vi "FFT.vi"() -> ()   [LabVIEW 2020]
uses:
  <vilib>/rvi/Analysis/measure/FFT/simModelSupport/niFPGA FFT Outside SCTL Sim Properties.ctl
  <vilib>/rvi/Analysis/measure/FFT/simModelSupport/niFPGA FFT Sim Types.ctl
  <vilib>/rvi/Analysis/measure/FFT/simModelSupport/niFpgaFFTSimArithmeticProperties.ctl
  <vilib>/rvi/Analysis/measure/FFT/simModelSupport/niFpgaFFTSimDfxp.ctl
  <vilib>/fxp/LVFixedPointQuantizationPolicyTypeDef.ctl
  <vilib>/rvi/FXPMathLib/FxpSinAndCos/subVIs/nifxpmath_SinAndCos_SimConfig.ctl
  <vilib>/rvi/DataTransferAndStorage/Container/Common/niFpgaContainerGetUniqueNameForEmu.vi
  <vilib>/rvi/DataTransferAndStorage/Container/Common/niFpgaContainerSetEmuInfo.vi
  <vilib>/rvi/eio/common/nirviEmuReportErrorAndStop.vi
  <vilib>/rvi/interface/RandomDataEmulation/niFpgaRandomDataHandleErrors.vi
  <vilib>/rvi/DataTransferAndStorage/Container/Common/niFpgaContainerExecOnDevCompGetState.vi
  <vilib>/rvi/Emulation/niFpgaEmulationIsFPGAContextNoSignature.vi
  <vilib>/rvi/Emulation/niFpgaSctlEmulationGetInTimedLoop.vi
  <vilib>/rvi/errors/niFpgaSetErrorForExecOnDevCompSimple.vi
  <vilib>/rvi/FIFO/Fifo_Resource/nirvififoEmulationSetSize.vi
  <vilib>/rvi/FIFO/Fifo_Resource/nirviFifoEmulationQueueMgr.vi
  <instcachedir>/0/nirviFifoEmulationQueueMgr_E5CAEC123FF24DC58D834DCA3CDAA9B5.lvgen/nirviFifoEmulationQueueMgr_E5CAEC123FF24DC58D834DCA3CDAA9B5_008.vi
  <vilib>/rvi/FIFO/Fifo_Resource/nirvififoEmulationDetermineInputValidOut.vi
  <vilib>/rvi/FIFO/Fifo_Resource/nirvififoEmulationCreateLock.vi
  <vilib>/rvi/Emulation/niFpgaProcessEmulError.vi
  <vilib>/rvi/FIFO/Fifo_Resource/nirvififoEmulationObtainLock.vi
  <vilib>/rvi/FIFO/Fifo_Resource/nirvififoEmulationReleaseLock.vi
  <vilib>/rvi/occurrence/nirviWaitOnOccurrenceBase.vi
  <vilib>/rvi/errors/nirviReportUnexpectedCaseInternalError.vi
  <vilib>/rvi/errors/nirviReportUnexpectedCaseInternalError (U32).vi
  <vilib>/Utility/error.llb/Clear Errors.vi
  <vilib>/rvi/Emulation/niFpgaGetClockAttributes.vi
  <vilib>/rvi/Emulation/niFpgaEmulationReportErrorSimple.vi
  <vilib>/rvi/Analysis/measure/FFT/simModelSupport/niFpgaFFTSimModelOutsideSCTLCore.vi
  <instcachedir>/0/nirviFifoEmulationQueueMgr_E5CAEC123FF24DC58D834DCA3CDAA9B5.lvgen/nirviFifoEmulationQueueMgr_E5CAEC123FF24DC58D834DCA3CDAA9B5_004.vi
  <vilib>/rvi/FXPMathLib/FxpSinAndCos/simVIs/DllFxpSinAndCosTemp_sub.vi
  <vilib>/rvi/Emulation/niFpgaCriticalErrorInLSC.vi
  <vilib>/rvi/LocalResourceManager/LocalResourceManager.xnode
  <vilib>/rvi/DataTransferAndStorage/Container/XNode/niFpgaContainer.xnode
  <vilib>/rvi/interface/RandomDataEmulation/nirviRandomDataFpgaReadWriteTemplate.vi
  <vilib>/rvi/FIFO/Fifo_Resource/niFpgaFifoEmulationRefIn.vi
  <vilib>/rvi/Analysis/measure/FFT/XNode/niFpgaFFT.xnode
  <vilib>/rvi/FXPMathLib/FxpSinAndCos/XNode/nifxpmath_SinAndCos.xnode
panel:
  out "Numeric 3":i32
  out "Numeric":i32
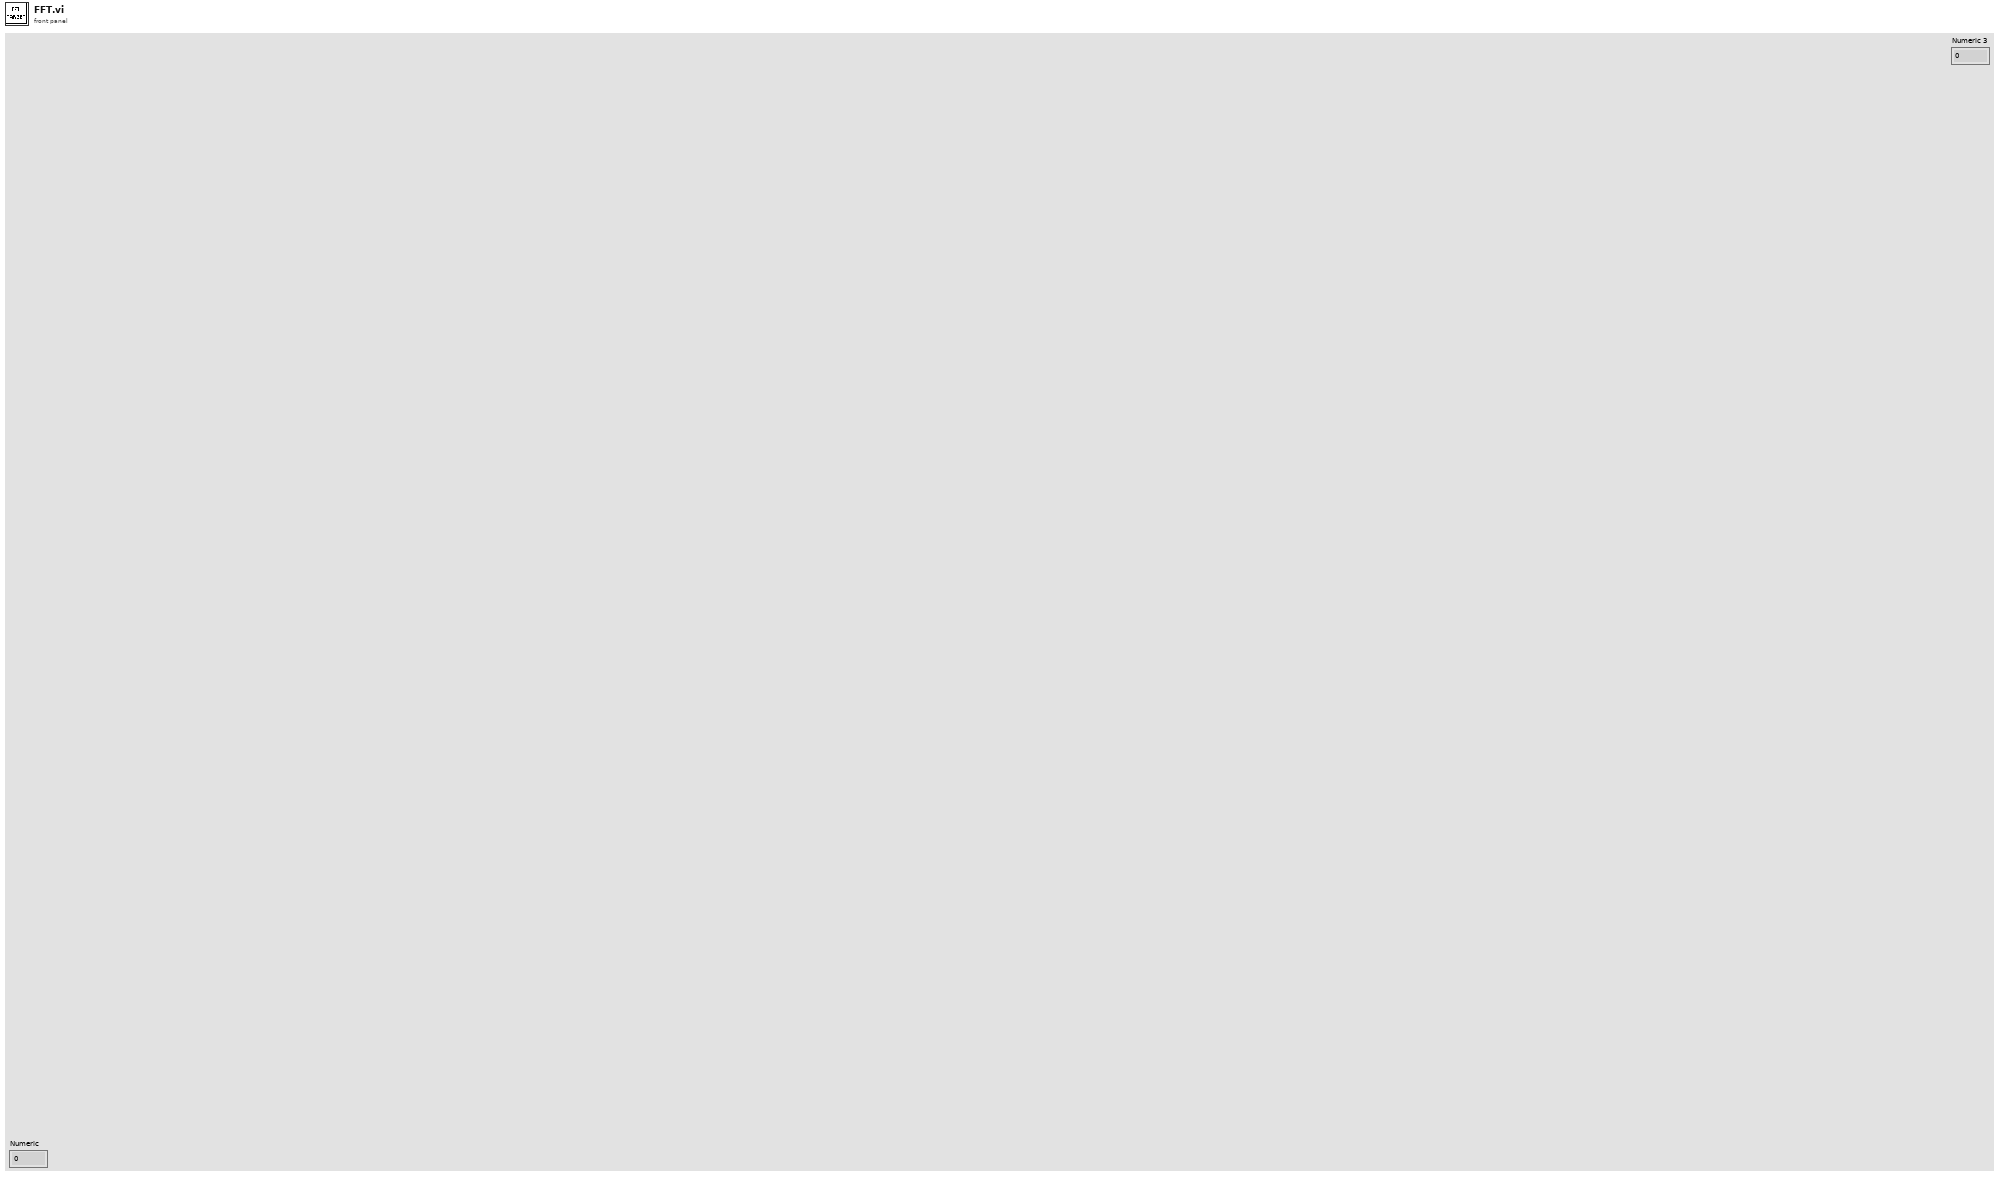
[diagram p1: front panel]
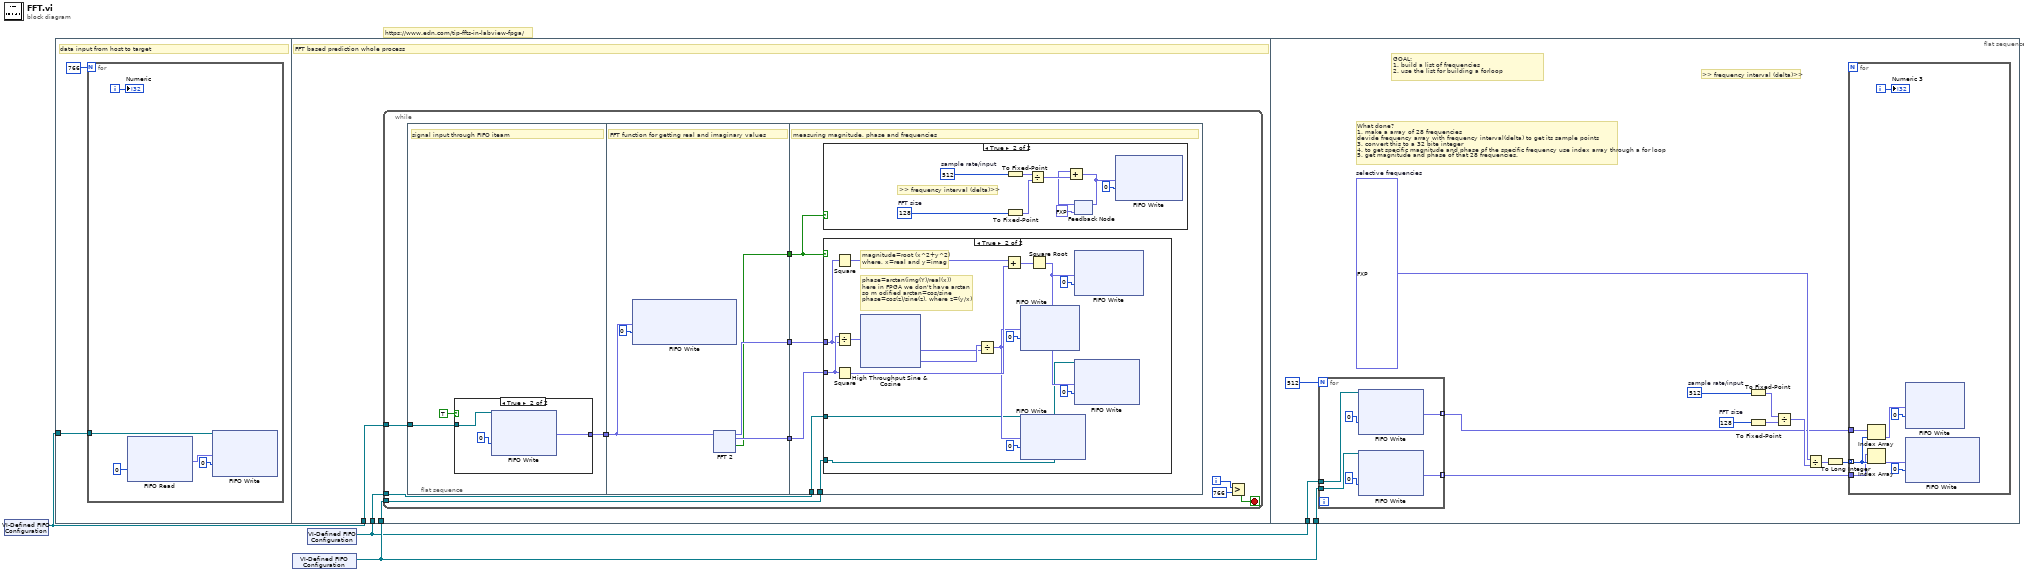
[diagram p0: block diagram]
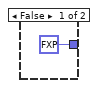
[diagram p2: hidden frame]
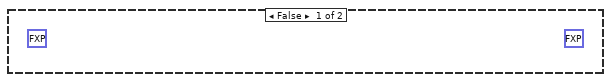
[diagram p4: hidden frame]
diagram:
  # "https://www.edn.com/tip-ffts-in-labview-fpga/"
  n1 = xnode "VI-Defined FIFO Configuration"() -> ("FIFO Out"=w3:refnum<k21>)
  n2 = flat-sequence {
    tunnel: w3 -> [w5]
    tunnel: w3 -> [w13]
    tunnel: w2 -> [w12]
    tunnel: w1 -> [w11]
    tunnel: w2 -> [w117]
    tunnel: w1 -> [w116]
    frame #0 {
      # "data input from host to target"
      n3 = for {
        N: 766 -> [_]
        tunnel: w5 -> [w9]
        i -> [w6]
        n4 = xnode ("FIFO Read")("Timeout"=0) -> ("Element"=w7:fxp<+/-,24,7>)  [unwired: 1 in, 2 out]
        n5 = xnode ("FIFO Write")("Element"=w7, "Timeout"=0, "FIFO In"=w9) -> ()  [unwired: 2 out]
        "Numeric" <- w6
      }
    }
    frame #1 {
      # "FFT based prediction whole process"
      n6 = while {
        tunnel: w13 -> [w22]
        tunnel: w12 -> [w15]
        tunnel: w11 -> [w14]
        i -> [w21]
        stop <- w16 stop-if-true
        n7 = flat-sequence {
          tunnel: w22 -> [w26]
          tunnel: [w24] -> w20
          tunnel: w20 -> [w35]
          tunnel: [w34] -> w19
          tunnel: [w33] -> w18
          tunnel: [w32] -> w17
          tunnel: w19 -> [w59]
          tunnel: w18 -> [w58]
          tunnel: w17 -> [w60]
          tunnel: w15 -> [w57]
          tunnel: w14 -> [w56]
          frame #0 {
            # "signal input through FIFO iteam"
            n8 = case shown="True" TRUE {
              tunnel: w26 -> [_ w30]
              tunnel: [fxp<+/-,24,7> 0.0 ("Element") w28] -> w24
              frame False {
              }
              frame True {
                n9 = xnode ("FIFO Write")("Timeout"=0, "FIFO In"=w30) -> ("Element"=w28:fxp<+/-,24,7>)  [unwired: 2 out]
              }
            }
          }
          frame #1 {
            # "FFT function for getting real and imaginary values"
            n10 = xnode ("FIFO Write")("Element"=w35, "Timeout"=0) -> ()  [unwired: 1 in, 2 out]
            n11 = xnode ("FFT 2")("real data in"=w35) -> ("real data out"=w34:fxp<+/-,32,15>, "imaginary data out"=w33:fxp<+/-,32,15>, "output valid"=w32:bool)  [unwired: 2 in, 1 out]
          }
          frame #2 {
            # "measuring magnitude, phase and frequencies"
            n12 = case shown="True" w60 {
              frame False {
              }
              frame True {
                w61 = 512  # sample rate/input
                w62 = 128  # FFT size
                # ">> frequency interval (delta)>>"
                n13 = To Fixed-Point(number=w61) -> (fixed-point=w64:fxp<+/-,32,32>)  [unwired: 1 in]
                n14 = To Fixed-Point(number=w62) -> (fixed-point=w63:fxp<+/-,32,32>)  [unwired: 1 in]
                n15 = Divide(x=w64, y=w63) -> (x/y=w68:fxp<+/-,32,16>)
                n16 = feedback #1(fxp<+/-,32,16> 0.0) -> (w66:fxp<+/-,32,16>)
                n17 = Add(x=w66, y=w68) -> (x+y=w67:fxp<+/-,32,16>)
                n18 = feedback-in #1(w67) -> ()
                n19 = xnode ("FIFO Write")("Element"=w67, "Timeout"=0) -> ()  [unwired: 1 in, 2 out]
              }
            }
            n20 = case shown="True" w60 {
              tunnel: w58 -> [_ w85]
              tunnel: w59 -> [_ w84]
              tunnel: w57 -> [_ w74]
              tunnel: w56 -> [_ w70]
              frame False {
                (unwired) fxp<+/-,32,16> 0.0
                (unwired) fxp<+/-,32,16> 0.0
              }
              frame True {
                # "magnitude=root (x^2+y^2)\nwhere, x=real and y=imag"
                # "phase=arctan(img(Y)/real(x))\nhere in FPGA we don't have arctan\nso m odified arctan=cos/sine\nphase=cos(z)/sine(z), where z=(y/x)"
                n21 = Square(x=w84) -> (x^2=w79:fxp<+,63,29>)
                n22 = Divide(x=w85, y=w84) -> (x/y=w77:fxp<+/-,32,16>)
                n23 = Square(x=w85) -> (x^2=w73:fxp<+,63,29>)
                n24 = xnode "High Throughput Sine & Cosine"("x (pi)"=w77) -> ("sin(x)"=w80:fxp<+/-,32,2>, "cos(x)"=w81:fxp<+/-,32,2>)
                n25 = Divide(x=w81, y=w80) -> (x/y=w72:fxp<+/-,32,16>)
                n26 = Add(x=w79, y=w73) -> (x+y=w78:fxp<+,64,30>)
                n27 = xnode ("FIFO Write")("Element"=w72, "Timeout"=0) -> ()  [unwired: 1 in, 2 out]
                n28 = xnode ("FIFO Write")("Element"=w72, "Timeout"=0, "FIFO In"=w70) -> ()  [unwired: 2 out]
                n29 = Square Root(x=w78) -> (sqrt(x)=w76:fxp<+/-,32,16>)
                n30 = xnode ("FIFO Write")("Element"=w76, "Timeout"=0) -> ()  [unwired: 1 in, 2 out]
                n31 = xnode ("FIFO Write")("Element"=w76, "Timeout"=0, "FIFO In"=w74) -> ()  [unwired: 2 out]
              }
            }
          }
        }
        n32 = Greater?(x=w21, y=766 ("Timeout")) -> (0:w16:bool)
      }
    }
    frame #2 {
      w122 = 512  # sample rate/input
      w123 = 128  # FFT size
      w124 = fxp<+/-,32,16>[] [128.0, 132.0, 136.0, 252.0, 256.0, 260.0, 380.0, 384.0, 388.0, -128.0, -132.0, -136.0, -252.0, -256.0, -260.0, -380.0, -384.0, -388.0]  # selective frequencies
      # "GOAL:\n1. build a list of frequencies\n2. use the list for building a forloop"
      # "What done?\n1. make a array of 28 frequencies\ndevide frequency array with frequency interval(delta) to get its sample points\n3. convert this to a 32 bite integer\n4. to get specific magnitude and phase of the specific frequency use index array through a for loop\n5. get magnitude and phase of that 28 frequencies."
      # ">> frequency interval (delta)>>"
      n33 = for {
        N: 512 -> [_]
        tunnel: [w140] -> w121 mode=indexing
        tunnel: [w139] -> w120 mode=indexing
        tunnel: w117 -> [w138]
        tunnel: w116 -> [w137]
        n34 = xnode ("FIFO Write")("Timeout"=0, "FIFO In"=w137) -> ("Element"=w140:fxp<+/-,32,16>)  [unwired: 2 out]
        n35 = xnode ("FIFO Write")("Timeout"=0, "FIFO In"=w138) -> ("Element"=w139:fxp<+/-,32,16>)  [unwired: 2 out]
      }
      n36 = To Fixed-Point(number=w122) -> (fixed-point=w126:fxp<+/-,32,32>)  [unwired: 1 in]
      n37 = To Fixed-Point(number=w123) -> (fixed-point=w125:fxp<+/-,32,32>)  [unwired: 1 in]
      n38 = Divide(x=w126, y=w125) -> (x/y=w127:fxp<+/-,32,16>)
      n39 = Divide(x=w124, y=w127) -> (x/y=w128:fxp<+/-,32,16>[])
      n40 = To Long Integer(number=w128) -> (32bit integer=w119:i32[])
      n41 = for {
        tunnel: w119 -> [w135] mode=indexing
        tunnel: w121 -> [w134]
        tunnel: w120 -> [w133]
        i -> [w136]
        n42 = Index Array(array=w134, index=w135) -> (element=w132:fxp<+/-,32,16>)
        n43 = Index Array(array=w133, index=w135) -> (element=w131:fxp<+/-,32,16>)
        n44 = xnode ("FIFO Write")("Element"=w132, "Timeout"=0) -> ()  [unwired: 1 in, 2 out]
        n45 = xnode ("FIFO Write")("Element"=w131, "Timeout"=0) -> ()  [unwired: 1 in, 2 out]
        "Numeric 3" <- w136
      }
    }
  }
  n46 = xnode "VI-Defined FIFO Configuration"() -> ("FIFO Out"=w2:refnum<k21>)
  n47 = xnode "VI-Defined FIFO Configuration"() -> ("FIFO Out"=w1:refnum<k21>)
